vi "Class to Variant.vi"(8 "error in (no error)":errorcluster, 10 "Data in":variant, 11 "Build Job in":refnum<class "Build Job.lvclass">) -> (0 "error out":errorcluster, 1 "Serialized Object Name":string, 2 "Data Out":variant, 3 "Build Job out":refnum<class "Build Job.lvclass">)   [LabVIEW 2014, in "Build Job.lvclass"]
uses:
  Build Job.lvclass
  Build Job.lvclass/Build Job.ctl
  Serializable Node/Serializable Node.lvclass
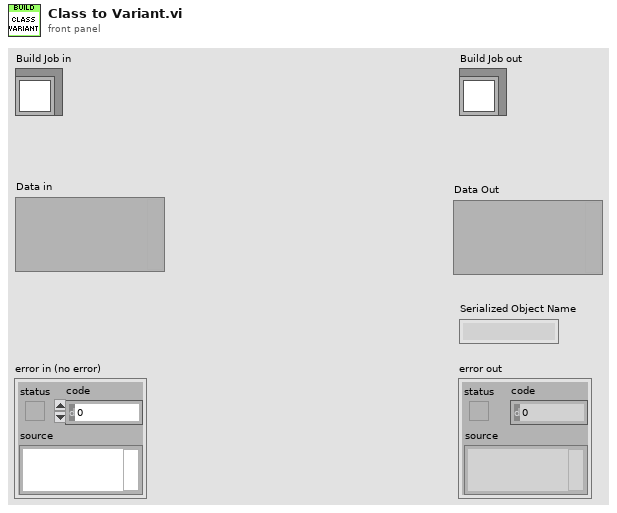
[diagram p1: front panel]
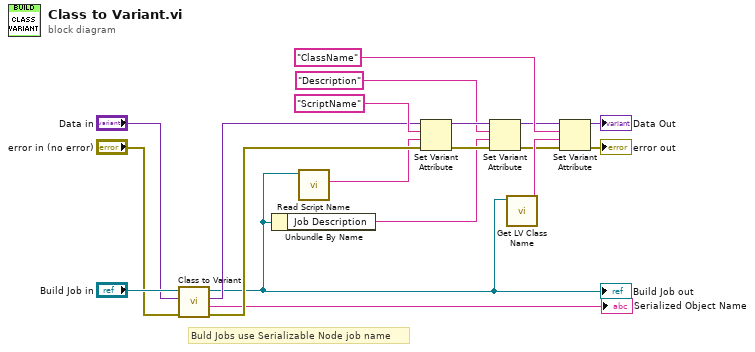
[diagram p0: block diagram]
diagram:
  # "Buld Jobs use Serializable Node job name"
  n1 = call-parent "Class to Variant.vi"("error in (no error)"="error in (no error)", "Data in"="Data in", "Serializable Node in"="Build Job in") -> ("error out"=w12:errorcluster, "Serialized Object Name"=→"Serialized Object Name":string, "Data Out"=w10:variant, "Serializable Node out"=w4:refnum<class "Build Job.lvclass">)  [unwired: 5 in]
  "Build Job out" <- w4
  n2 = Unbundle By Name(w4) -> ("Job Description"=w14:string)
  n3 = call-dynamic "Read Script Name.vi"("Build Job in"=w4) -> ("Script Name"=w9:string)  [unwired: 10 in]
  n4 = Set Variant Attribute(Variant=w10, name="ScriptName", value=w9, error in=w12) -> (Variant out=w18:variant, error out=w17:errorcluster)  [unwired: 1 out]
  n5 = Set Variant Attribute(Variant=w18, name="Description", value=w14, error in=w17) -> (Variant out=w6:variant, error out=w5:errorcluster)  [unwired: 1 out]
  n6 = call <vilib>:"Get LV Class Name.vi"("object"=w4) -> ("class name"=w8:string)  [unwired: 9 in, 1 out]
  n7 = Set Variant Attribute(Variant=w6, name="ClassName", value=w8, error in=w5) -> (Variant out=→"Data Out":variant, error out=→"error out":errorcluster)  [unwired: 1 out]
